vi "filenameparser_09.vi"(6 "Description":string, 7 "start path":path=path "", 9 "Project name":string, 10 "User (initials)":string, 11 "OK Button in":bool) -> (1 "Output file":string, 2 "appended path 2":path, 3 "appended path":path)   [LabVIEW 2016]
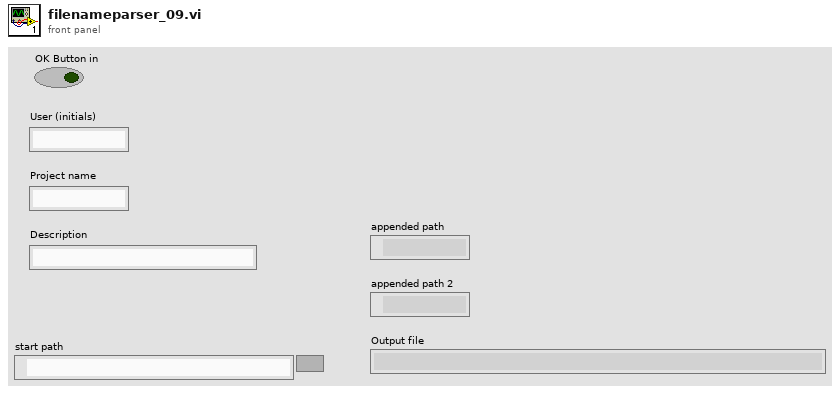
[diagram p1: front panel]
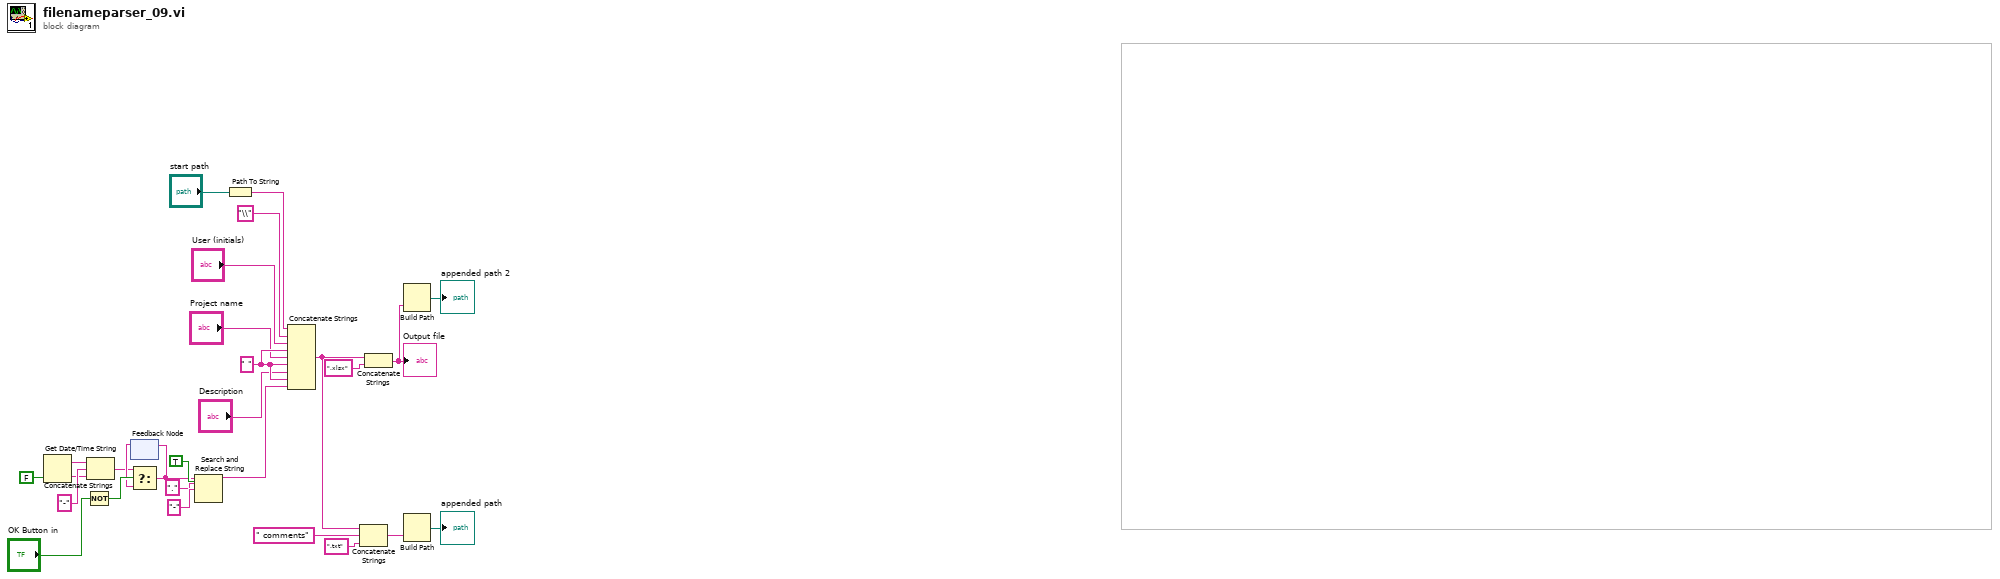
[diagram p0: block diagram]
diagram:
  w7 = " "
  n1 = Get Date/Time String(want seconds? (F)=FALSE) -> (date string=w10:string, time string=w15:string)  [unwired: 2 in]
  n2 = Not(x="OK Button in") -> (.not. x?=w14:bool)
  n3 = Concatenate Strings(w10, "-" ("string"), w15) -> (w11:string)
  n4 = feedback #1() -> (w12:string)  [unwired: 1 in]
  n5 = Select(t=w11, s=w14, f=w12) -> (s? t:f=w19:string)
  n6 = feedback-in #1(w19) -> ()
  n7 = Search and Replace String(replace all?=TRUE ("replace all? (F)"), input string=w19, search string=".", replace string="-" ("replace string (\"\")")) -> (result string=w20:string)  [unwired: 4 in, 3 out]
  n8 = Path To String(path="start path") -> (string=w2:string)
  n9 = Concatenate Strings(w2, "\\" ("string"), "User (initials)", w7, "Project name", w7, "Description", w7, w20) -> (w24:string)
  n10 = Concatenate Strings(w24, " comments" ("string"), ".txt" ("string")) -> (w27:string)
  n11 = Concatenate Strings(w24, ".xlsx") -> (w22:string)
  "Output file" <- w22
  n12 = Build Path(name or relative path=w22) -> (appended path=→"appended path 2":path)  [unwired: 1 in]
  n13 = Build Path(name or relative path=w27) -> (appended path=→"appended path":path)  [unwired: 1 in]
